vi "BLM MoveAndWait.vi"(1 "Mode IS:":bool, 2 "Steps/rot":dbl=8000.0, 3 "error in (no error)":errorcluster, 4 "Position / Distance":dbl=1.0 min=-193273528.32 max=193273528.0 step=0.09 format="%.2f", 5 "Motor Address":string="0", 6 "Instrument Address":refnum<visa-resource-name>) -> (0 "error out":errorcluster)   [LabVIEW 2016]
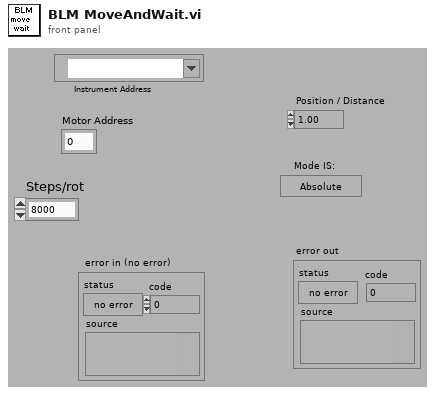
[diagram p1: front panel]
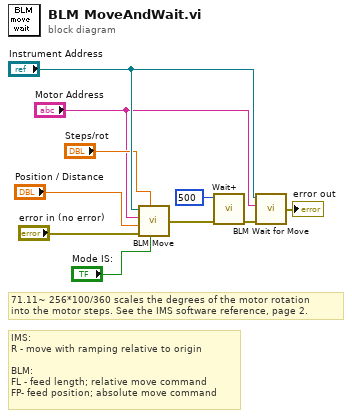
[diagram p0: block diagram]
diagram:
  # "IMS:\nR - move with ramping relative to origin\n\nBLM:\nFL - feed length; relative move command\nFP- feed position; absolute move command"
  # "71.11~ 256*100/360 scales the degrees of the motor rotation\ninto the motor steps. See the IMS software reference, page 2."
  n1 = call "BLM Move.vi"("Mode IS:"="Mode IS:", "Steps/rot"="Steps/rot", "error in (no error)"="error in (no error)", "Position / Distance"="Position / Distance", "Motor Address"="Motor Address", "Port Address"="Instrument Address") -> ("error out"=w10:errorcluster)
  n2 = call "Wait+.vi"("Error In"=w10, "milliseconds to wait"=u32 500) -> ("Error Out"=w9:errorcluster)  [unwired: 4 in, 1 out]
  n3 = call "BLM Wait for Move.vi"("PORT Address"="Instrument Address", "Motor Address"="Motor Address", "error in (no error)"=w9) -> ("error out"=→"error out":errorcluster)  [unwired: 2 in]
